vi "ExposeExtractVariantValueAndDeleteRefrence.vi"(10 "Delete Refrence? (T)":bool=TRUE, 11 "Data Value Reference in":refnum<data-value>) -> (3 "Value out":variant)   [LabVIEW 2017]
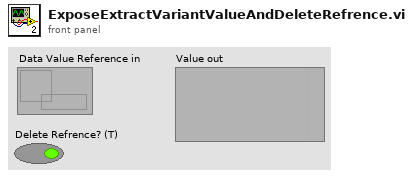
[diagram p1: front panel]
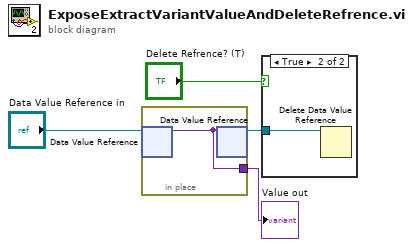
[diagram p0: block diagram]
diagram:
  n1 = in-place {
    in-place-border: [w5] -> w4
    n2 = in-place-dvr #1("Data Value Reference in") -> (w5:variant)  [unwired: 1 out]
    n3 = in-place-dvr #1(w5) -> (w3:refnum<data-value>)  [unwired: 1 out]
  }
  "Value out" <- w4
  n4 = case shown="True" "Delete Refrence? (T)" {
    tunnel: w3 -> [_ w6]
    frame False {
    }
    frame True {
      n5 = Delete Data Value Reference(data value reference=w6) -> ()  [unwired: 1 in, 2 out]
    }
  }
